vi "ADIS16470 RefNum Registry Get.vi"(8 "error in (no error)":errorcluster, 10 "refnum name":string="My IMU RefNum") -> (0 "error out":errorcluster, 3 "ADIS16470DevRef out":T1={"DevStatus"={"status"=FALSE, "code"=0, "source"=""}, "Hardware Config"={"SPI Clock Rate (Hz)"=1000000.0, "IMU SPI Mode (3)"=enum."Mode 3 (Clk Idle High,Sample on Trailing)", "IMU Reset Pin"=enum."SPI Port CS2", "IMU SPI Bus"=enum."SPI On-Board, CS0", "IMU Data Ready Pin"=enum."SPI Port CS1", "Stall Config"={"Pow2BytesPerRead"=255, "StallTicks"=640, "CsToSclkTicks"=5}}, "Calibration Complete"=refnum, "Status Reference"=refnum, "Position Reference"=refnum, "Velocity Reference"=refnum, "Sychronous Process VI"=refnum, "Cmd FIFO"=refnum, "Source"={"DevStatus"={"status"=FALSE, "code"=0, "source"=""}, "AnalogTriggerMode?"=FALSE, "DigitalMode"={"DIO Channel"=enum."Disabled"}, "AnalogTriggerMode"={"AnalogTriggerIndex"=enum."Trig 0", "OutputType"=enum."InWindow"}}, "Data FIFO"=refnum, "Calibration Time (ms)"=5})   [LabVIEW 2020]
doc: "Gets the reference you specify. You first must set the reference with the RefNum Registry Set VI."
uses:
  Typedef/ADIS16470 Device Reference.ctl
  Typedef/ADIS16470 Hardware Configuration.ctl
  <vilib>/Rock Robotics/WPI/SPI/WPI_SPIMode.ctl
  <vilib>/Rock Robotics/SystemInterfaces/DIO/FPGA_DIOChannel.ctl
  <vilib>/Rock Robotics/SystemInterfaces/spilib/spi_bus.ctl
  Typedef/ADIS16470 Status.ctl
  Typedef/ADIS16470 Data.ctl
  Typedef/ADIS16470 Process.ctl
  Typedef/ADIS16470 Command Type.ctl
  <vilib>/Rock Robotics/SystemInterfaces/CounterEncoderSourceConvertion/FPGA_CounterEncoderSourceConvertionLVSourceType.ctl
  <vilib>/Rock Robotics/SystemInterfaces/DIO/FPGA_DIODigitalSourceChannel.ctl
  <vilib>/Rock Robotics/SystemInterfaces/AnalogTrigger/FPGA_AnalogTriggerIndex.ctl
  <vilib>/Rock Robotics/SystemInterfaces/AnalogTrigger/FPGA_AnalogTriggerOutType.ctl
  <vilib>/Rock Robotics/WPI/Utilities/Refnum Registry Operation.ctl
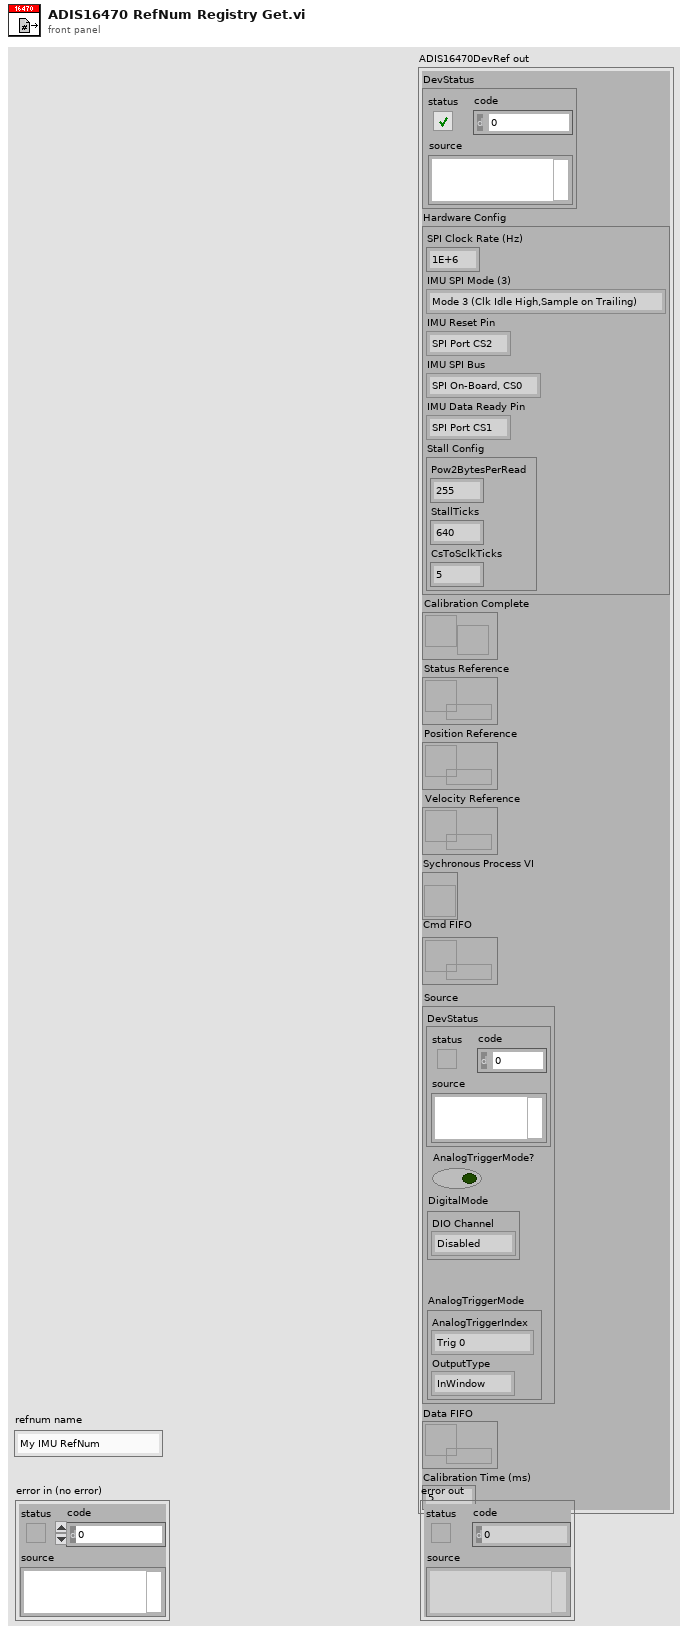
[diagram p1: front panel]
types:
  T1 = typedef "ADIS16470 Device Reference.ctl" = cluster{"DevStatus":errorcluster, "Hardware Config":T2, "Calibration Complete":refnum<notifier>, "Status Reference":refnum<data-value>, "Position Reference":refnum<data-value>, "Velocity Reference":refnum<data-value>, "Sychronous Process VI":T6, "Cmd FIFO":refnum<k33>, "Source":T7, "Data FIFO":refnum<k33>, "Calibration Time (ms)":u32}
  T2 = typedef "ADIS16470 Hardware Configuration.ctl" = cluster{"SPI Clock Rate (Hz)":dbl, "IMU SPI Mode (3)":T3, "IMU Reset Pin":T4, "IMU SPI Bus":T5, "IMU Data Ready Pin":T4, "Stall Config":cluster{"Pow2BytesPerRead":u8, "StallTicks":u16, "CsToSclkTicks":u8}}
  T3 = typedef "WPI_SPIMode.ctl" = enum16{"Mode 0 (Clk Idle Low,Sample on Leading)", "Mode 1 (Clk Idle Low,Sample on Trailing)", "Mode 2 (Clk Idle High,Sample on Leading)", "Mode 3 (Clk Idle High,Sample on Trailing)"}
  T4 = typedef "FPGA_DIOChannel.ctl" = enum8{"DIO 0", "DIO 1", "DIO 2", "DIO 3", "DIO 4", "DIO 5", "DIO 6", "DIO 7", "DIO 8", "DIO 9", "DIO MXP 0", "DIO MXP 1", "DIO MXP 2", "DIO MXP 3", "DIO MXP 4", "DIO MXP 5", "DIO MXP 6", "DIO MXP 7", "DIO MXP 8", "DIO MXP 9", "DIO MXP 10", "DIO MXP 11", "DIO MXP 12", "DIO MXP 13", "DIO MXP 14", "DIO MXP 15", "SPI Port CS1", "SPI Port CS2", "SPI Port CS3", "SPI Port MISO", "SPI Port MOSI", "Invalid"}
  T5 = typedef "spi_bus.ctl" = enum16{"SPI On-Board, CS0", "SPI On-Board, CS1", "SPI On-Board, CS2", "SPI On-Board, CS3", "SPI MXP", "Invalid"}
  T6 = typedef "ADIS16470 Process.ctl" = refnum<vi>
  T7 = typedef "FPGA_CounterEncoderSourceConvertionLVSourceType.ctl" = cluster{"DevStatus":errorcluster, "AnalogTriggerMode?":bool, "DigitalMode":cluster{"DIO Channel":T8}, "AnalogTriggerMode":cluster{"AnalogTriggerIndex":T9, "OutputType":T10}}
  T8 = typedef "FPGA_DIODigitalSourceChannel.ctl" = enum8{"DIO 0", "DIO 1", "DIO 2", "DIO 3", "DIO 4", "DIO 5", "DIO 6", "DIO 7", "DIO 8", "DIO 9", "DIO MXP 0", "DIO MXP 1", "DIO MXP 2", "DIO MXP 3", "DIO MXP 4", "DIO MXP 5", "DIO MXP 6", "DIO MXP 7", "DIO MXP 8", "DIO MXP 9", "DIO MXP 10", "DIO MXP 11", "DIO MXP 12", "DIO MXP 13", "DIO MXP 14", "DIO MXP 15", "SPI Port CS1", "SPI Port CS2", "SPI Port CS3", "SPI Port MISO", "SPI Port MOSI", "Disabled"}
  T9 = typedef "FPGA_AnalogTriggerIndex.ctl" = enum8{"Trig 0", "Trig 1", "Trig 2", "Trig 3", "Trig 4", "Trig 5", "Trig 6", "Trig 7", "Invalid"}
  T10 = typedef "FPGA_AnalogTriggerOutType.ctl" = enum16{"InWindow", "TriggerState", "Rising", "Falling"}
  T11 = typedef "Refnum Registry Operation.ctl" = enum16{"set", "get", "delete", "get all names", "read name"}
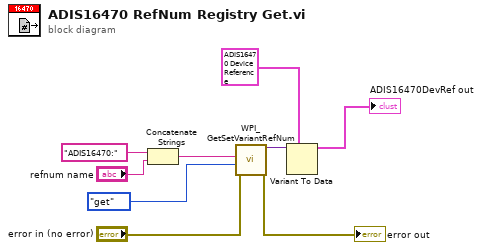
[diagram p0: block diagram]
diagram:
  n1 = Concatenate Strings("ADIS16470:", "refnum name") -> (w9:string)
  n2 = call <vilib>:"WPI_GetSetVariantRefNum.vi"("error in (no error)"="error in (no error)", "Operation"=Refnum_Registry_Operation."get" ("menu"), "refnum name"=w9) -> ("error out"=→"error out":errorcluster, "DevRef"=w7:variant)  [unwired: 6 in, 1 out]
  n3 = Variant To Data(type=T1 {"DevStatus"={"status"=FALSE, "code"=0, "source"=""}, "Hardware Config"={"SPI Clock Rate (Hz)"=1000000.0, "IMU SPI Mode (3)"=enum."Mode 3 (Clk Idle High,Sample on Trailing)", "IMU Reset Pin"=enum."SPI Port CS2", "IMU SPI Bus"=enum."SPI On-Board, CS0", "IMU Data Ready Pin"=enum."SPI Port CS1", "Stall Config"={"Pow2BytesPerRead"=255, "StallTicks"=640, "CsToSclkTicks"=5}}, "Calibration Complete"=refnum, "Status Reference"=refnum, "Position Reference"=refnum, "Velocity Reference"=refnum, "Sychronous Process VI"=refnum, "Cmd FIFO"=refnum, "Source"={"DevStatus"={"status"=FALSE, "code"=0, "source"=""}, "AnalogTriggerMode?"=FALSE, "DigitalMode"={"DIO Channel"=enum."Disabled"}, "AnalogTriggerMode"={"AnalogTriggerIndex"=enum."Trig 0", "OutputType"=enum."InWindow"}}, "Data FIFO"=refnum, "Calibration Time (ms)"=5} ("ADIS16470DevRef in"), Variant=w7) -> (data=→"ADIS16470DevRef out":T1)  [unwired: 1 in, 1 out]
